vi "CIC_5decimate_1cycle_32_bit_for_5761.vi"(7 "reset":bool, 8 "valid in":bool, 11 "Data in":fxp<+/-,32,14>) -> (0 "valid out":bool, 3 "Data out":fxp<+/-,32,14>)   [LabVIEW 2018]
uses:
  <vilib>/rvi/FXPMathLib/FxpConvert/subVIs/nifxpmath_Convert_SimConfig.ctl
  <vilib>/fxp/LVFixedPointQuantizationPolicyTypeDef.ctl
  <vilib>/fxp/LVFixedPointOverflowPolicyTypeDef.ctl
  <vilib>/rvi/IPIntegrationNode/IPINode_Typedef/niFpgaIPINodeSupportedFamilies.ctl
  <vilib>/rvi/FXPMathLib/FxpConvert/simVIs/DllFxpConvertTemp_sub.vi
  <vilib>/rvi/IPIntegrationNode/IPINode_Utilities/niFpgaIPINodeSimCore.vi
  <vilib>/rvi/FXPMathLib/FxpInterpret/XNode/nifxpmath_Interpret.xnode
  <vilib>/rvi/FXPMathLib/FxpMul/XNode/nifxpmath_Multiplier.xnode
  <vilib>/rvi/FXPMathLib/FxpConvert/XNode/nifxpmath_Convert.xnode
  <vilib>/rvi/XilinxIP/XIPIN_XNode/niFpgaXIPIN.xnode
  CIC_5decimate_1cycle_32_bit_for_5761/xsim.dir/CIC_5decimate_1cycle_32_bit_for_5761_418948D8E56E498F91A60A22D0632EB3/xsimk_418948D8E56E498F91A60A22D0632EB3.dll
  <vilib>/rvi/IPIntegrationNode/IPINode_Xnode/niFpgaIPINode.xnode
  <vilib>/rvi/FXPMathLib/sim/FxpSim.dll
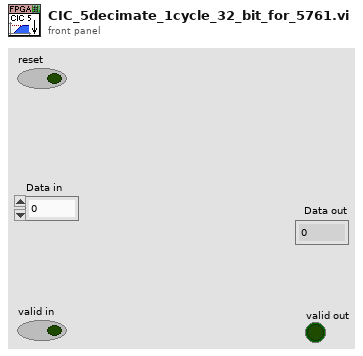
[diagram p1: front panel]
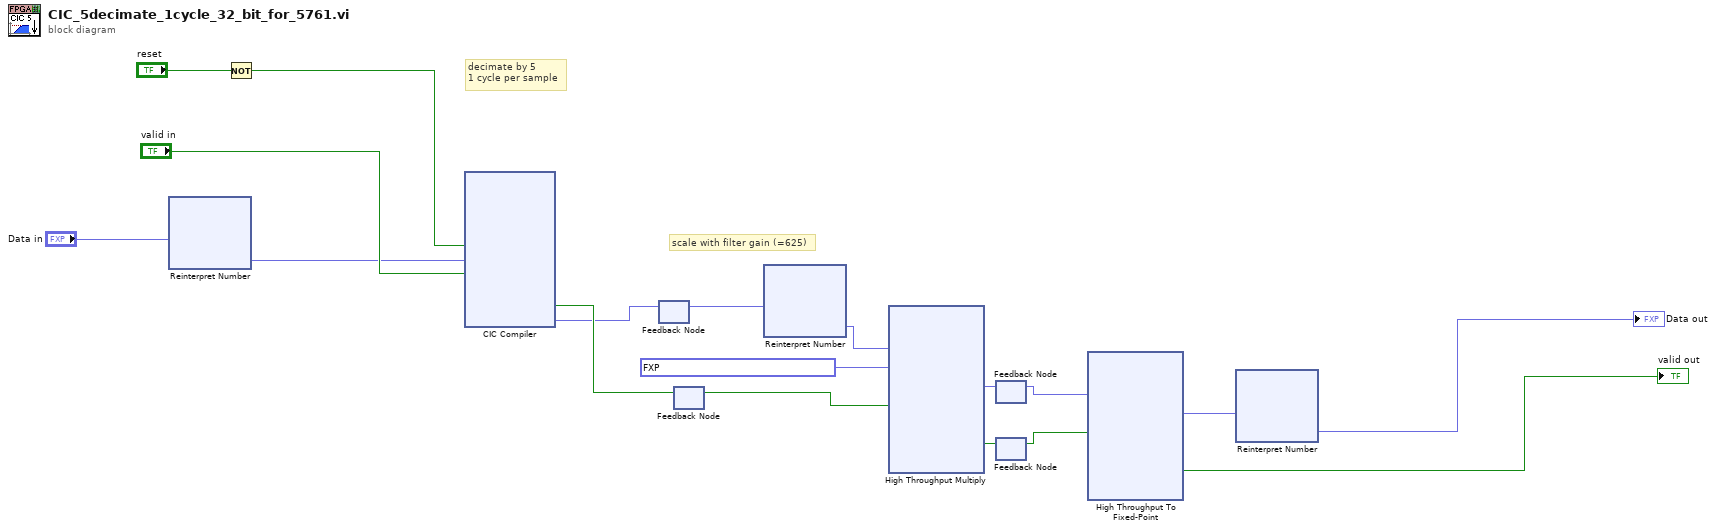
[diagram p0: block diagram]
diagram:
  # "scale with filter gain (=625)"
  # "decimate by 5\n1 cycle per sample"
  n1 = xnode "Reinterpret Number"("x"="Data in") -> ("y"=w3:fxp<+,32,32>)
  n2 = Not(x="reset") -> (.not. x?=w5:bool)
  n3 = xnode ("CIC Compiler")("aresetn"=w5, "s_axis_data_tdata"=w3, "s_axis_data_tvalid"="valid in") -> ("m_axis_data_tvalid"=w2:bool, "m_axis_data_tdata"=w1:fxp<+,48,48>)  [unwired: 1 in, 1 out]
  n4 = feedback #1() -> (w13:fxp<+,48,48>)  [unwired: 1 in]
  n5 = feedback-in #1(w1) -> ()
  n6 = feedback #2() -> (w14:bool)  [unwired: 1 in]
  n7 = feedback-in #2(w2) -> ()
  n8 = xnode "Reinterpret Number"("x"=w13) -> ("y"=w12:fxp<+/-,48,48>)
  n9 = xnode ("High Throughput Multiply")("x"=w12, "y"=fxp<+/-,32,1> 0.001600000075995922, "input valid"=w14) -> ("x*y"=w16:fxp<+/-,64,49>, "output valid"=w17:bool)  [unwired: 1 in, 1 out]
  n10 = feedback #3() -> (w10:fxp<+/-,64,49>)  [unwired: 1 in]
  n11 = feedback-in #3(w16) -> ()
  n12 = feedback #4() -> (w9:bool)  [unwired: 1 in]
  n13 = feedback-in #4(w17) -> ()
  n14 = xnode "High Throughput To Fixed-Point"("x"=w10, "input valid"=w9) -> ("y"=w11:fxp<+/-,32,32>, "output valid"=→"valid out":bool)  [unwired: 1 in, 1 out]
  n15 = xnode "Reinterpret Number"("x"=w11) -> ("y"=→"Data out":fxp<+/-,32,14>)
